vi "Global FPGA.vi"() -> ()   [LabVIEW 2015]
panel:
  out "PPS":bool
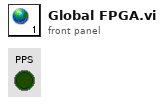
[diagram p1: front panel]
diagram:
